vi "mupExpr sglExpr sglVar with constants example.vi"() -> ()   [LabVIEW 2015]
uses:
  mupExpr/mupExpr.lvclass
  mupExpr/mupExpr.lvclass/mupExpr.ctl
  mupExpr/Eval_SglVar_SglRes.vi
  mupExpr/Read Singe Var Name.vi
  mupLib/mupEval.vi
  mupLib/mupSetVarValue.vi
  mupLib/mupCheckError.vi
  mupLib/mupLibPath.vi
  <vilib>/Utility/error.llb/Error Cluster From Error Code.vi
panel:
  out "Variable Name":string
  out "Variable Values":dbl[](array[numeric])
  out "Results":dbl[](array[numeric])
  in  "Constants":cluster{"name":string, "value":dbl}[](array[cluster])=[{"name"="a", "value"=1.0}, {"name"="b", "value"=2.0}, {"name"="c", "value"=3.0}]
  out "error out":errorcluster
  in  "Expression":string="a*x^2+b*x+c"
  # "This example demonstrates the basic usage of mupExpr. It will evaluate the input expression assuming a\nsingle variable with values from 0 to 9. If more than one variable is used, the result will be NaN.\n\n- Enter an expression composed up to one variable\n- Enter the constant names and values that may be used by the expression\n- Hit run to evaluate the expression for variable values of 0 to 9"
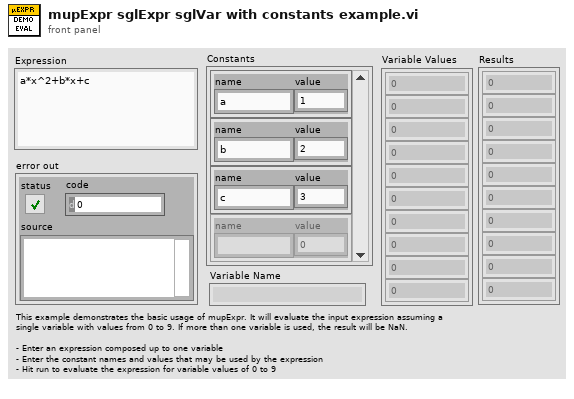
[diagram p1: front panel]
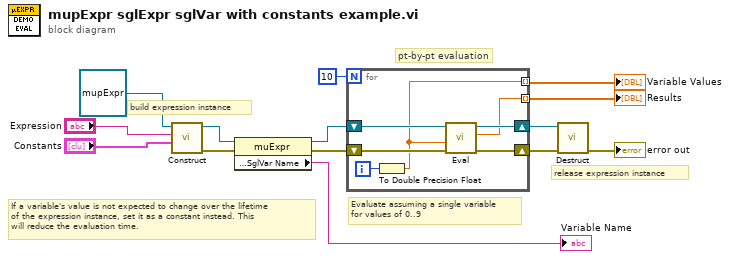
[diagram p0: block diagram]
diagram:
  # "If a variable's value is not expected to change over the lifetime\nof the expression instance, set it as a constant instead. This\nwill reduce the evaluation time."
  # "pt-by-pt evaluation"
  # "release expression instance"
  # "build expression instance"
  # "Evaluate assuming a single variable\nfor values of 0..9"
  n1 = call-dynamic "Construct.vi"("Constants"="Constants", "Expression"="Expression", "muExpr in"=refnum<class "mupExpr.lvclass"> refnum) -> ("error out"=w3:errorcluster, "mupExpr out"=w6:refnum<class "mupExpr.lvclass">)  [unwired: 5 in, 2 out]
  n2 = property class="muExpr"(reference=w6, error in=w3) -> (reference out=w5:refnum<class "mupExpr.lvclass">, error out=w2:errorcluster, "Properties:SglVar Name"=→"Variable Name":string)
  n3 = for {
    N: 10 -> [_]
    shift-right: [w18] -> w13
    shift-left: w5 -> [w20]
    shift-right: [w17] -> w12
    shift-left: w2 -> [w19]
    tunnel: [w16] -> w8 mode=indexing
    tunnel: [w15] -> w7 mode=indexing
    i -> [w21]
    n4 = To Double Precision Float(number=w21) -> (double precision float=w15:dbl)
    n5 = call-poly "Eval.vi"("error in (no error)"=w19, "varValue"=w15, "muExpr in"=w20) -> ("error out"=w17:errorcluster, "Result"=w16:dbl, "muExpr out"=w18:refnum<class "mupExpr.lvclass">)  [unwired: 6 in]
  }
  "Results" <- w8
  "Variable Values" <- w7
  n6 = call-dynamic "Destruct.vi"("error in (no error)"=w12, "muExpr in"=w13) -> ("error out"=→"error out":errorcluster)  [unwired: 9 in]
